vi "Query Operation Complete.vi"(8 "error in (no error)":errorcluster, 10 "Capture Mode (0: Scan)":u32(ring) items=["Scan", "Trigger"], 11 "VISA resource name":refnum<visa-resource-name>) -> (0 "error out":errorcluster, 2 "Complete":bool, 3 "VISA resource name out":refnum<visa-resource-name>)   [LabVIEW 2023, in "Keithley DMM6500 DAQ6500 Series.lvlib"]
doc: "Reads and returns the state of the present scan/trigger, the scan/trigger count, and the step count."
uses:
  <instrlib>/Keithley DMM6500 DAQ6500 Series/Keithley DMM6500 DAQ6500 Series.lvlib
  <vilib>/regexp/Match Regular Expression.xnode
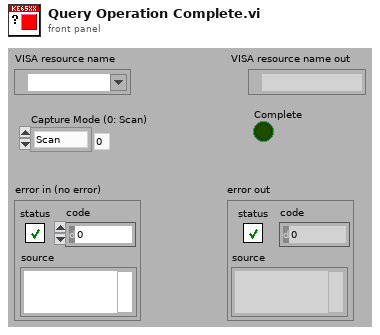
[diagram p1: front panel]
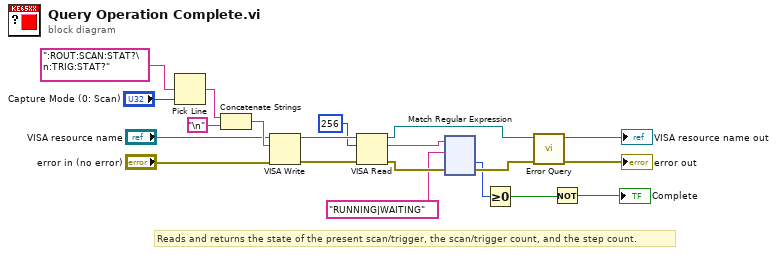
[diagram p0: block diagram]
diagram:
  # "Reads and returns the state of the present scan/trigger, the scan/trigger count, and the step count."
  n1 = Pick Line(multi-line string=":ROUT:SCAN:STAT?\n:TRIG:STAT?", line index="Capture Mode (0: Scan)") -> (output string=w10:string)  [unwired: 1 in]
  n2 = Concatenate Strings(w10, "\n") -> (w20:string)
  n3 = VISA Write(VISA resource name="VISA resource name", write buffer=w20, error in (no error)="error in (no error)") -> (VISA resource name out=w16:refnum<visa-resource-name>, error out=w15:errorcluster)  [unwired: 1 out]
  n4 = VISA Read(VISA resource name=w16, byte count=u32 256, error in (no error)=w15) -> (VISA resource name out=w11:refnum<visa-resource-name>, read buffer=w6:string, error out=w8:errorcluster)  [unwired: 1 out]
  n5 = xnode "Match Regular Expression"("input string"=w6, "regular expression"="RUNNING|WAITING", "error in"=w8) -> ("offset past match"=w3:i32, "error out"=w7:errorcluster)  [unwired: 3 in, 3 out]
  n6 = Greater Or Equal To 0?(x=w3) -> (x >= 0?=w2:bool)
  n7 = call <instrlib>:"Error Query.vi"("error in (no error)"=w7, "VISA resource name"=w11) -> ("error out"=→"error out":errorcluster, "VISA resource name out"=→"VISA resource name out":refnum<visa-resource-name>)  [unwired: 6 in, 2 out]
  n8 = Not(x=w2) -> (.not. x?=→"Complete":bool)
